vi "set_triggered.vi"(8 "error in (no error)":errorcluster, 10 "triggered?":bool, 11 "FPGA_AK101022Resonance in":refnum<class "FPGAWrapperAK101022Resonance.lvclass">) -> (0 "error out":errorcluster, 3 "FPGA_AK101022Resonance out":refnum<class "FPGAWrapperAK101022Resonance.lvclass">)   [LabVIEW 2010]
uses:
  FPGAWrapperAK101022Resonance.lvclass
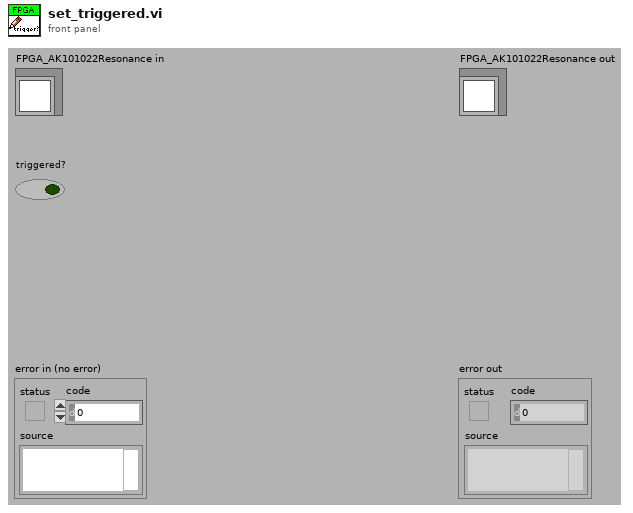
[diagram p1: front panel]
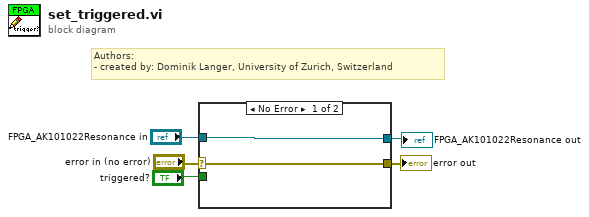
[diagram p0: block diagram]
diagram:
  # "Authors: \n- created by: Dominik Langer, University of Zurich, Switzerland"
  n1 = case shown="No Error" "error in (no error)" {
    selector: "error in (no error)" -> [w7 w8]
    tunnel: "triggered?" -> [_ _]
    tunnel: "FPGA_AK101022Resonance in" -> [w6 w9]
    tunnel: [w6 w9] -> w2
    tunnel: [w7 w8] -> w5
    frame No Error {
    }
    frame Error {
    }
  }
  "error out" <- w5
  "FPGA_AK101022Resonance out" <- w2
